vi "loadImages.vi"(9 "BGImages":T1, 10 "Numeric":i32=2, 11 "data":T3) -> (1 "time":u32, 2 "BG Images out":T1, 3 "dat6a out":T3)   [LabVIEW 2020]
uses:
  analysis_data_typdef.ctl
  IMAQ Image.ctl
  bgImages_tyudef.ctl
  MagAnalysis_Online.lvclass
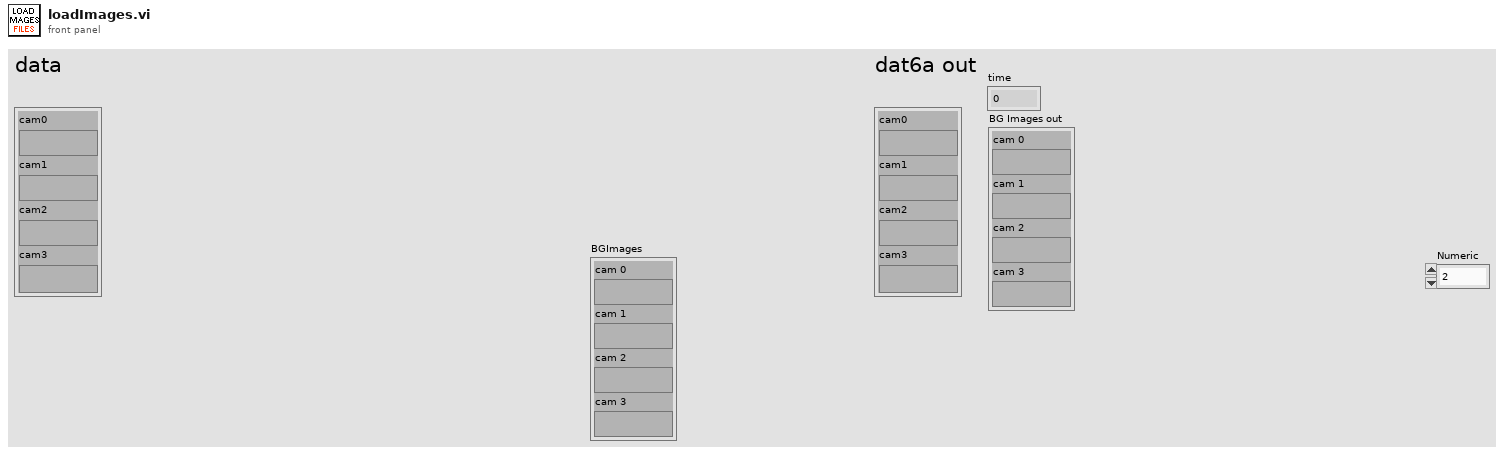
[diagram p1: front panel]
types:
  T1 = typedef "bgImages_tyudef.ctl" = cluster{"cam 0":T2, "cam 1":T2, "cam 2":T2, "cam 3":T2}
  T2 = typedef "IMAQ Image.ctl" = refnum<image>
  T3 = typedef "MagAnalysis_Online.lvclass/analysis_data_typdef.ctl" = cluster{"cam0":T2, "cam1":T2, "cam2":T2, "cam3":T2}
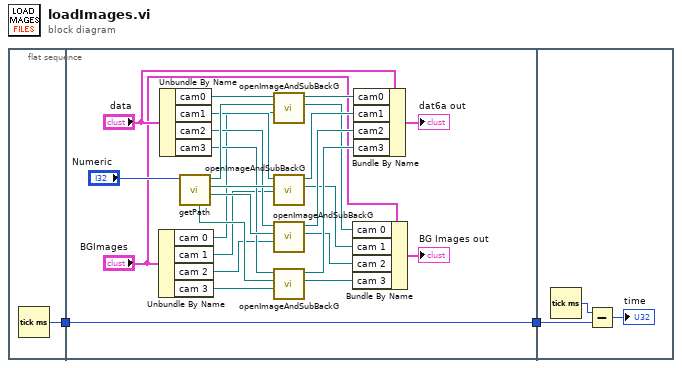
[diagram p0: block diagram]
diagram:
  n1 = flat-sequence {
    tunnel: [w3] -> w2
    tunnel: w2 -> [w14]
    tunnel: [w14] -> w1
    tunnel: w1 -> [w31]
    frame #0 {
      n2 = Tick Count (ms)() -> (millisecond timer value=w3:u32)
    }
    frame #1 {
      n3 = Unbundle By Name("BGImages") -> ("cam 0"=w7:T2, "cam 1"=w6:T2, "cam 2"=w5:T2, "cam 3"=w4:T2)
      n4 = Unbundle By Name("data") -> ("cam0"=w21:T2, "cam1"=w27:T2, "cam2"=w25:T2, "cam3"=w22:T2)
      n5 = call "getPath.vi"("Numeric"="Numeric") -> ("cam2"=w24:path, "cam1"=w26:path, "cam0"=w28:path, "cam3"=w23:path)  [unwired: 7 in]
      n6 = call "openImageAndSubBackG.vi"("BG image"=w7, "image in"=w28, "image"=w21) -> ("BG Out"=w13:T2, "raw Image out"=w19:T2)  [unwired: 7 in]
      n7 = call "openImageAndSubBackG.vi"("BG image"=w6, "image in"=w26, "image"=w27) -> ("BG Out"=w12:T2, "raw Image out"=w18:T2)  [unwired: 7 in]
      n8 = call "openImageAndSubBackG.vi"("BG image"=w5, "image in"=w24, "image"=w25) -> ("BG Out"=w11:T2, "raw Image out"=w17:T2)  [unwired: 7 in]
      n9 = call "openImageAndSubBackG.vi"("BG image"=w4, "image in"=w23, "image"=w22) -> ("BG Out"=w10:T2, "raw Image out"=w16:T2)  [unwired: 7 in]
      n10 = Bundle By Name(cluster="BGImages", "cam 0"=w13, "cam 1"=w12, "cam 2"=w11, "cam 3"=w10) -> (→"BG Images out":T1)
      n11 = Bundle By Name(cluster="data", "cam0"=w19, "cam1"=w18, "cam2"=w17, "cam3"=w16) -> (→"dat6a out":T3)
    }
    frame #2 {
      n12 = Tick Count (ms)() -> (millisecond timer value=w32:u32)
      n13 = Subtract(x=w32, y=w31) -> (x-y=→"time":u32)
    }
  }
